vi "6 bytes to parsing.vi"(11 "Output data format":T2(ring)) -> (2 "data packet length":i32, 3 "First 6 bytes":T1)   [LabVIEW 2017, in "IL Driver Library.lvlib"]
uses:
  IL Driver Library.lvlib
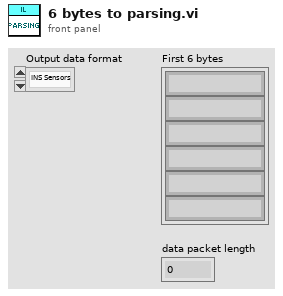
[diagram p1: front panel]
types:
  T1 = cluster{string, string, string, string, string, string}
  T2 = enum16{"INS Sensors", "INS OPVT", "INS QPVT", "INS OPVT2A", "INS OPVT2AW", "INS OPVT2Ahr", "INS Minimal", "INS NMEA"}
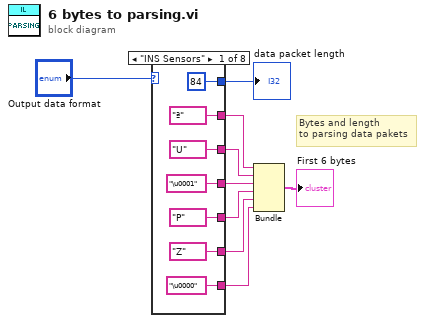
[diagram p0: block diagram]
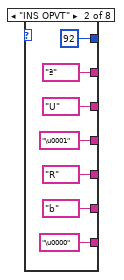
[diagram p2: hidden frame]
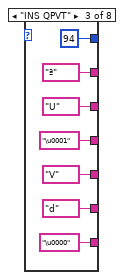
[diagram p3: hidden frame]
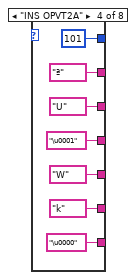
[diagram p4: hidden frame]
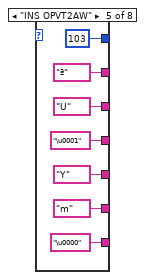
[diagram p5: hidden frame]
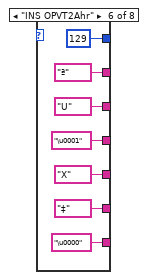
[diagram p6: hidden frame]
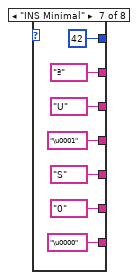
[diagram p7: hidden frame]
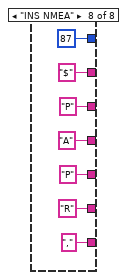
[diagram p8: hidden frame]
diagram:
  # "Bytes and length\nto parsing data pakets"
  n1 = case shown="\"INS Sensors\"" "Output data format" {
    tunnel: [84 ("y") 92 ("y") 94 ("y") 101 ("y") 103 ("y") 129 ("y") 42 ("y") 87 ("y")] -> w1
    tunnel: ["ª" "ª" "ª" "ª" "ª" "ª" "ª" "$"] -> w2
    tunnel: ["U" "U" "U" "U" "U" "U" "U" "P"] -> w3
    tunnel: ["\u0001" "\u0001" "\u0001" "\u0001" "\u0001" "\u0001" "\u0001" "A"] -> w4
    tunnel: ["P" "R" "V" "W" "Y" "X" "S" "P"] -> w5
    tunnel: ["Z" "b" "d" "k" "m" "‡" "0" "R"] -> w6
    tunnel: ["\u0000" "\u0000" "\u0000" "\u0000" "\u0000" "\u0000" "\u0000" ","] -> w7
    frame "INS Sensors" {
    }
    frame "INS OPVT" {
    }
    frame "INS QPVT" {
    }
    frame "INS OPVT2A" {
    }
    frame "INS OPVT2AW" {
    }
    frame "INS OPVT2Ahr" {
    }
    frame "INS Minimal" {
    }
    frame "INS NMEA" {
    }
  }
  "data packet length" <- w1
  n2 = Bundle(w2, w3, w4, w5, w6, w7) -> (→"First 6 bytes":T1)  [unwired: 1 in]
